vi "MGCC_FntStaMach_flag_solver.vi"   [LabVIEW 2016]
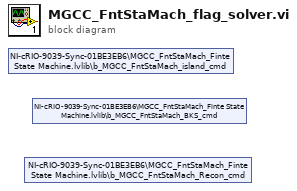
[diagram p0: block diagram]
diagram:
  n1 = shared-variable "NI-cRIO-9039-Sync-01BE3EB6\\MGCC_FntStaMach_Finte State Machine.lvlib\\b_MGCC_FntStaMach_island_cmd"() -> ()  [unwired: 1 in, 2 out]
  n2 = shared-variable "NI-cRIO-9039-Sync-01BE3EB6\\MGCC_FntStaMach_Finte State Machine.lvlib\\b_MGCC_FntStaMach_Recon_cmd"() -> ()  [unwired: 1 in, 2 out]
  n3 = shared-variable "NI-cRIO-9039-Sync-01BE3EB6\\MGCC_FntStaMach_Finte State Machine.lvlib\\b_MGCC_FntStaMach_BKS_cmd"() -> ()  [unwired: 1 in, 2 out]
